vi "app_pktParse.vi"(11 "pkts_get":string[](array[string])) -> (0 "total_pkts":u32, 3 "app_pkt":T1(array[cluster]))   [LabVIEW 2014]
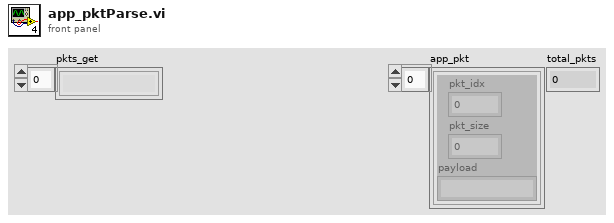
[diagram p1: front panel]
types:
  T1 = cluster{"pkt_idx":u32, "pkt_size":u32, "payload":string}[]
  T2 = cluster{"pkt_idx":u32, "pkt_size":u32, "payload":string}
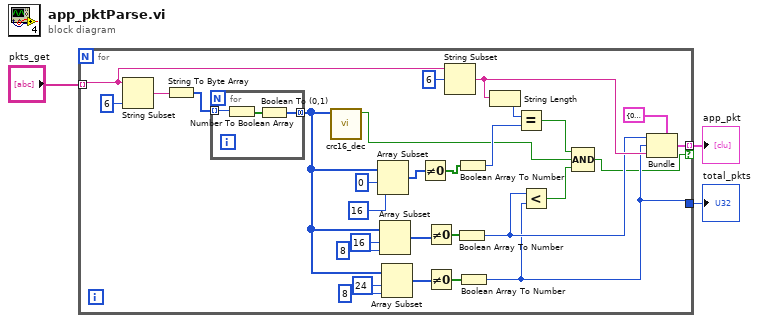
[diagram p0: block diagram]
diagram:
  n1 = for {
    tunnel: "pkts_get" -> [w19] mode=indexing
    tunnel: [w13] -> w2 mode=indexing if=w4
    tunnel: [w8] -> w1
    n2 = String Subset(string=w19, length (rest)=6 ("length (rest)")) -> (substring=w31:string)  [unwired: 1 in]
    n3 = String To Byte Array(string=w31) -> (unsigned byte array=w30:u8[])
    n4 = for {
      tunnel: w30 -> [w35] mode=indexing
      tunnel: [w33] -> w29 mode=concatenating
      n5 = Number To Boolean Array(number=w35) -> (Boolean array=w34:bool[])
      n6 = Boolean To (0,1)(Boolean=w34) -> (0, 1=w33:i16[])
    }
    n7 = call "crc16_dec.vi"("Bit and crc16"=w29) -> ("passed"=w6:bool)  [unwired: 10 in]
    n8 = Array Subset(array=w29, index=0, length=16) -> (w20:i16[])
    n9 = Array Subset(array=w29, index=16, length=8) -> (w21:i16[])
    n10 = Array Subset(array=w29, index=24, length=8) -> (w22:i16[])
    n11 = Not Equal To 0?(x=w20) -> (x != 0?=w17:bool[])
    n12 = Not Equal To 0?(x=w21) -> (x != 0?=w16:bool[])
    n13 = Not Equal To 0?(x=w22) -> (x != 0?=w15:bool[])
    n14 = String Subset(string=w19, offset (0)=6) -> (substring=w12:string)  [unwired: 1 in]
    n15 = Boolean Array To Number(Boolean array=w16) -> (number=w9:u32)
    n16 = Boolean Array To Number(Boolean array=w17) -> (number=w10:u32)
    n17 = Boolean Array To Number(Boolean array=w15) -> (number=w8:u32)
    n18 = String Length(string=w12) -> (length=w11:i32)
    n19 = Equal?(x=w11, y=w10) -> (x = y?=w7:bool)
    n20 = Less?(x=w9, y=w8) -> (x < y?=w5:bool)
    n21 = Compound Arithmetic op=AND(w7, w6, w5) -> (w4:bool)
    n22 = Bundle(cluster=T2 {"pkt_idx"=0, "pkt_size"=0, "payload"=""}, "pkt_idx"=w9, "pkt_size"=w8, "payload"=w12) -> (w13:T2)
  }
  "app_pkt" <- w2
  "total_pkts" <- w1
